vi "Read Status Line(s).vi"(11 "httpResponse in":refnum<class "httpResponse.lvclass">) -> (2 "status line":string, 3 "httpResponse dup":refnum<class "httpResponse.lvclass">)   [LabVIEW 2020, in "httpClient.lvlib" / "httpResponse.lvclass"]
uses:
  httpResponse.lvclass
  httpResponse.lvclass/httpResponse.ctl
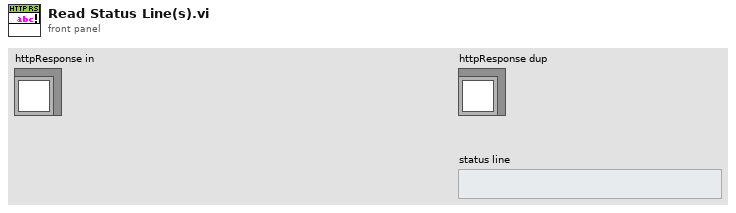
[diagram p1: front panel]
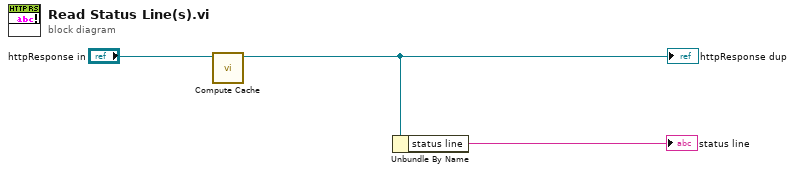
[diagram p0: block diagram]
diagram:
  n1 = call "Compute Cache.vi"("httpResponse in"="httpResponse in") -> ("httpResponse out"=w1:refnum<class "httpResponse.lvclass">)  [unwired: 9 in, 1 out]
  "httpResponse dup" <- w1
  n2 = Unbundle By Name(w1) -> ("status line"=→"status line":string)
